vi "TopLevel.vi"() -> ()   [LabVIEW 2011]
uses:
  <vilib>/FPGAPlugInAG/cRIO-9113/niLvFpga_Open_cRIO-9113.vi
  2-Think/2 Globals/2 Global.vi
  <vilib>/Utility/error.llb/Error Cluster From Error Code.vi
  <vilib>/rvi/errors/niLvFpgaAdjustHostInterfaceError.vi
  <vilib>/FPGAPlugInAG/cRIO-9113/niLvFpga_Close_cRIO-9113.vi
  <vilib>/rvi/interface/nirviOpenFPGA/nirviOpenFPGA.xnode
  FPGA Bitfiles/SailBot_FPGATarget_FPGA_CB0D9804.lvbitx
  FPGA/FPGA.vi
  <vilib>/rvi/interface/nirviReadWriteControl/nirviReadWriteControl.xnode
  <vilib>/rvi/interface/nirviCloseFPGA/nirviCloseFPGA.xnode
  NiFpgaLv.dll
panel:
  in  "stop":bool
  out "error out":errorcluster
  # "Winch"
  # "Rudder"
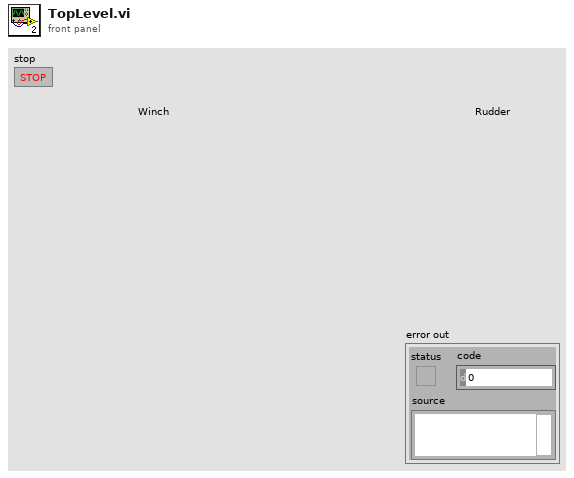
[diagram p1: front panel]
types:
  T1 = typedef "rudder angle.ctl" = dbl
  T2 = typedef "sail setpt.ctl" = dbl
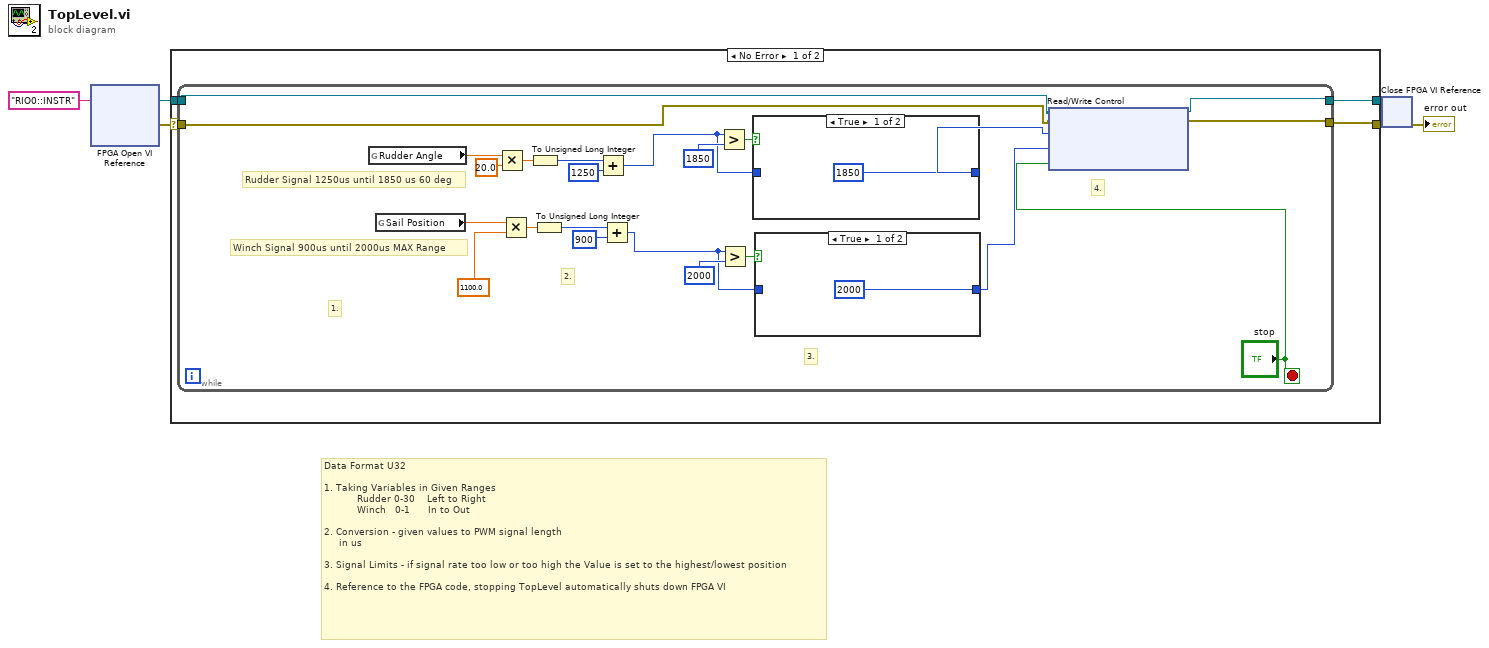
[diagram p0: block diagram]
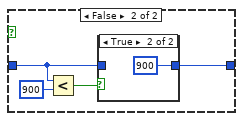
[diagram p2: hidden frame]
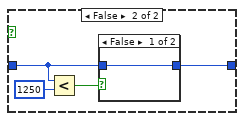
[diagram p4: hidden frame]
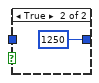
[diagram p5: hidden frame]
diagram:
  # "Data Format U32\n\n1. Taking Variables in Given Ranges\n           Rudder 0-30    Left to Right\n           Winch   0-1      In to Out\n\n2. Conversion - given values to PWM signal length\n     in us\n\n3. Signal Limits - if signal rate too low or too high the Value is set to the highest/lowest position\n\n4. Reference to the FPGA code, stopping TopLevel automatically shuts down FPGA VI"
  n1 = xnode "FPGA Open VI Reference"("resource name"="RIO0::INSTR") -> ("FPGA VI Reference Out"=w4:refnum<k20>, "error out"=w3:errorcluster)  [unwired: 1 in]
  n2 = case shown="No Error" w3 {
    selector: w3 -> [w10 w48]
    tunnel: [w7 w49] -> w2
    tunnel: [w8 w48] -> w1
    tunnel: w4 -> [w9 w49]
    frame No Error {
      n3 = while {
        tunnel: w9 -> [w22]
        tunnel: w10 -> [w23]
        tunnel: [w21] -> w8
        tunnel: [w20] -> w7
        stop <- "stop" stop-if-true
        # "4."
        # "3."
        # "2."
        # "1."
        # "Winch Signal 900us until 2000us MAX Range"
        # "Rudder Signal 1250us until 1850 us 60 deg"
        n4 = global read "2 Global.vi" "Rudder Angle"() -> (w12:T1)
        n5 = global read "2 Global.vi" "Sail Position"() -> (w11:T2)
        n6 = Multiply(x=w12, y=20.0) -> (x*y=w32:T1)
        n7 = Multiply(x=w11, y=1100.0) -> (x*y=w28:T2)
        n8 = To Unsigned Long Integer(number=w32) -> (unsigned 32bit integer=w31:u32)
        n9 = To Unsigned Long Integer(number=w28) -> (unsigned 32bit integer=w27:u32)
        n10 = Add(x=w31, y=u32 1250) -> (x+y=w14:u32)
        n11 = Add(x=w27, y=u32 900) -> (x+y=w13:u32)
        n12 = Greater?(x=w14, y=u32 1850 ("upper limit")) -> (0:w24:bool)
        n13 = Greater?(x=w13, y=u32 2000 ("upper limit")) -> (0:w17:bool)
        n14 = case shown="True" w24 {
          tunnel: w14 -> [_ w43]
          tunnel: [u32 1850 ("upper limit") w42] -> w19
          frame True {
          }
          frame False {
            n15 = Less?(x=w43, y=1250 ("lower limit")) -> (x < y?=w44:bool)
            n16 = case shown="False" w44 {
              tunnel: [w46 1250 ("upper limit")] -> w42
              tunnel: w43 -> [w46 _]
              frame False {
              }
              frame True {
              }
            }
          }
        }
        n17 = case shown="True" w17 {
          tunnel: w13 -> [_ w36]
          tunnel: [2000 ("upper limit") w35] -> w16
          frame True {
          }
          frame False {
            n18 = Less?(x=w36, y=900 ("lower limit")) -> (x < y?=w37:bool)
            n19 = case shown="True" w37 {
              tunnel: [w39 900 ("upper limit")] -> w35
              tunnel: w36 -> [w39 _]
              frame False {
              }
              frame True {
              }
            }
          }
        }
        n20 = xnode "Read/Write Control"("FPGA VI Reference In"=w22, "error in"=w23, "SERVO 2 Duty in Ticks"=w19, "SERVO 1 Duty in Ticks"=w16, "stop PWM"="stop") -> ("FPGA VI Reference Out"=w20:refnum<k20>, "error out"=w21:errorcluster)
      }
    }
    frame Error {
      # "Error occurred. Do not run."
    }
  }
  n21 = xnode "Close FPGA VI Reference"("FPGA VI Reference In"=w2, "error in"=w1) -> ("error out"=→"error out":errorcluster)
